vi "Get Build Spec Info.vi"(8 "error in":errorcluster caption="Error In", 10 "Build Spec Name":string, 11 "Project Path":path) -> (0 "sortie d'erreur":errorcluster caption="Error Out", 3 "VI Ref":refnum<vi>)   [LabVIEW 2015]
doc: "Open the VI reference pointed by the VI Name input. This function does not require a path as input but requires that the VI is present in the same project as the calling VI."
panel:
  out "Nom":string
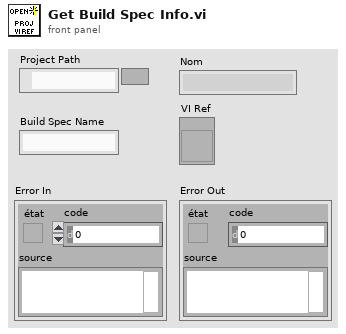
[diagram p1: front panel]
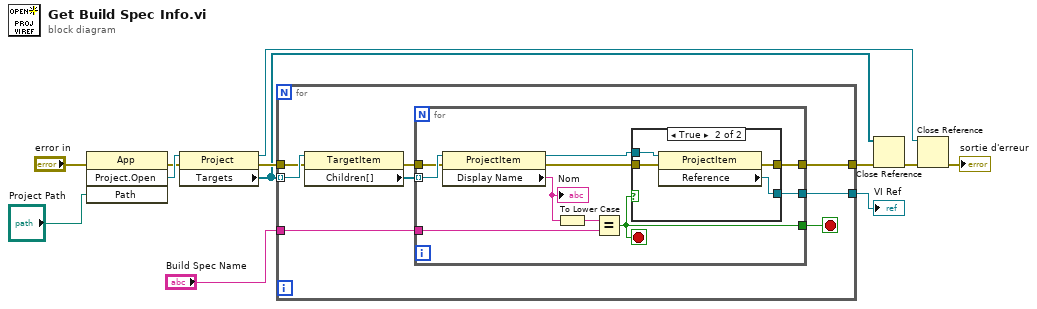
[diagram p0: block diagram]
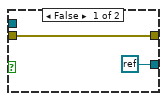
[diagram p2: hidden frame]
diagram:
  n1 = invoke class="App" method="Project.Open"(error in="error in", "Path"="Project Path") -> (error out=w3:errorcluster, "Project:Open"=w4:refnum<vi>)  [unwired: 2 in, 2 out]
  n2 = property class="Project"(reference=w4, error in=w3) -> (reference out=w2:refnum<vi>, error out=w12:errorcluster, "Targets"=w8:refnum<vi>[])
  n3 = for {
    tunnel: w8 -> [w20] mode=indexing
    tunnel: w12 -> [w18]
    tunnel: [w15] -> w11
    tunnel: [w14] -> w10
    tunnel: "Build Spec Name" -> [w13]
    stop <- w16 stop-if-true
    n4 = property class="TargetItem"(reference=w20, error in=w18) -> (error out=w17:errorcluster, "Children[]"=w19:refnum<vi>[])  [unwired: 1 out]
    n5 = for {
      tunnel: w19 -> [w30] mode=indexing
      tunnel: w17 -> [w28]
      tunnel: [w25] -> w16
      tunnel: [w24] -> w15
      tunnel: [w23] -> w14
      tunnel: w13 -> [w22]
      stop <- w25 stop-if-true
      n6 = property class="ProjectItem"(reference=w30, error in=w28) -> (reference out=w27:refnum<vi>, error out=w26:errorcluster, "Display Name"=w29:string)
      "Nom" <- w29
      n7 = To Lower Case(string=w29) -> (all lower case string=w21:string)
      n8 = Equal?(x=w21, y=w22) -> (x = y?=w25:bool)
      n9 = case shown="True" w25 {
        tunnel: w27 -> [_ w36]
        tunnel: w26 -> [w31 w35]
        tunnel: [refnum<k0> refnum w34] -> w24
        tunnel: [w31 w33] -> w23
        frame False {
        }
        frame True {
          n10 = property class="ProjectItem"(reference=w36, error in=w35) -> (error out=w33:errorcluster, "Reference"=w34:refnum<vi>)  [unwired: 1 out]
        }
      }
    }
  }
  "VI Ref" <- w11
  n11 = Close Reference(reference=w8, error in (no error)=w10) -> (error out=w9:errorcluster)
  n12 = Close Reference(reference=w2, error in (no error)=w9) -> (error out=→"sortie d'erreur":errorcluster)
